vi "EJEM17.vi"() -> ()   [LabVIEW 2013]
panel:
  out "element":dbl
  out "subarray 2":dbl[](array[numeric])
  out "subarray":dbl[](array[numeric])
  out "appended array 3":dbl[](array[numeric])
  out "appended array 2":dbl[](array[numeric])
  out "appended array":dbl[](array[numeric])
  out "initialized array":dbl[](array[numeric])
  out "size(s)":i32
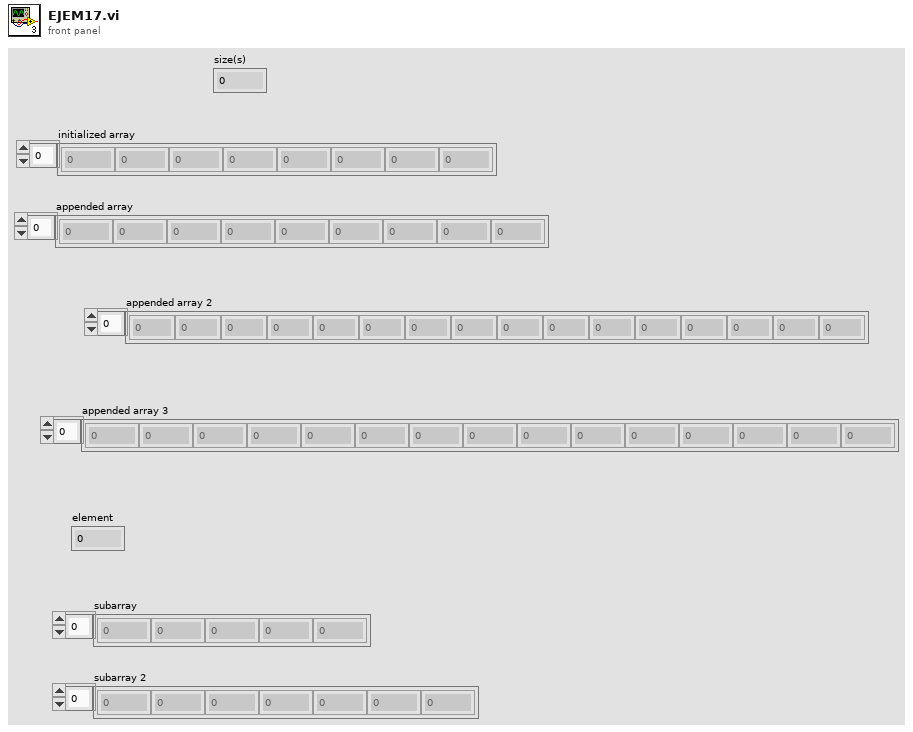
[diagram p1: front panel]
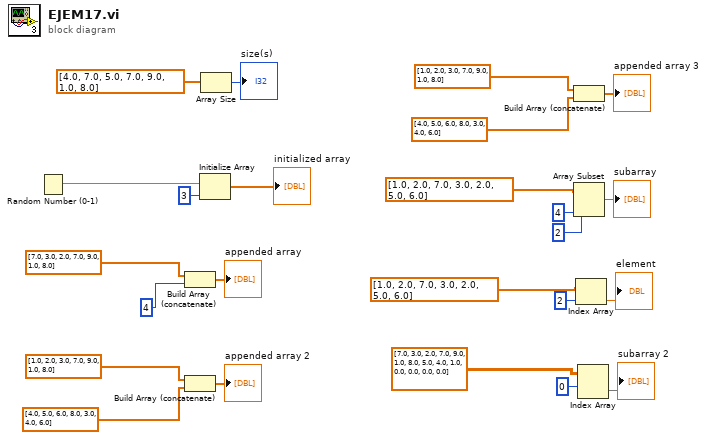
[diagram p0: block diagram]
diagram:
  n1 = Random Number (0-1)() -> (number: 0 to 1=w22:dbl)
  n2 = Build Array (concatenate)(dbl[] [7.0, 3.0, 2.0, 7.0, 9.0, 1.0, 8.0] ("array"), 4) -> (→"appended array":dbl[])
  n3 = Build Array (concatenate)(dbl[] [1.0, 2.0, 3.0, 7.0, 9.0, 1.0, 8.0] ("array"), dbl[] [4.0, 5.0, 6.0, 8.0, 3.0, 4.0, 6.0] ("array")) -> (→"appended array 2":dbl[])
  n4 = Initialize Array(w22, 3 ("dimension size")) -> (→"initialized array":dbl[])
  n5 = Array Size(array=dbl[] [4.0, 7.0, 5.0, 7.0, 9.0, 1.0, 8.0]) -> (size(s)=→"size(s)":i32)
  n6 = Build Array (concatenate)(dbl[] [1.0, 2.0, 3.0, 7.0, 9.0, 1.0, 8.0] ("array"), dbl[] [4.0, 5.0, 6.0, 8.0, 3.0, 4.0, 6.0] ("array")) -> (→"appended array 3":dbl[])
  n7 = Array Subset(array=dbl[] [1.0, 2.0, 7.0, 3.0, 2.0, 5.0, 6.0], index=2, length=4) -> (→"subarray":dbl[])
  n8 = Index Array(array=dbl[] [1.0, 2.0, 7.0, 3.0, 2.0, 5.0, 6.0], index=2) -> (element=→"element":dbl)
  n9 = Index Array(array=dbl[][] [[7.0, 3.0, 2.0, 7.0, 9.0, 1.0, 8.0], [5.0, 4.0, 1.0, 0.0, 0.0, 0.0, 0.0]], index (row)=0 ("index")) -> (element=→"subarray 2":dbl[])  [unwired: 1 in]
